vi "Set New Product.vi"(6 "error in (no error)":errorcluster, 9 "Cluster":T1) -> (0 "error out":errorcluster, 3 "success?":bool)   [LabVIEW 2020, in "SQLITE Inventory.lvlib"]
uses:
  SQLITE Inventory.lvlib
  Invetory Data Type.ctl
  <vilib>/drjdpowell/SQLite Library/SQL Connection/Open (path).vi
  <vilib>/drjdpowell/SQLite Library/SQL Connection/Open (string).vi
  <vilib>/AdvancedString/Path To Command Line String.vi
  <vilib>/drjdpowell/SQLite Library/SQL Connection/Execute SQL (No results).vi
  <vilib>/drjdpowell/SQLite Library/SQL Connection/Connection.lvclass
  <vilib>/drjdpowell/SQLite Library/SQLite.lvlib
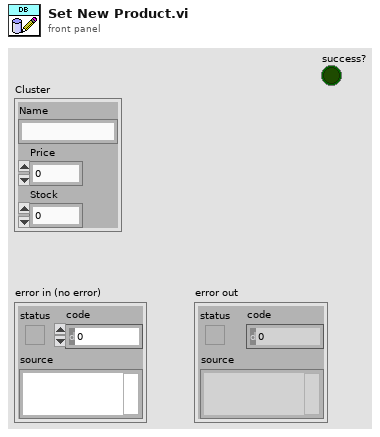
[diagram p1: front panel]
types:
  T1 = typedef "Invetory Data Type.ctl" = cluster{"Name":string, "Price":dbl, "Stock":dbl}
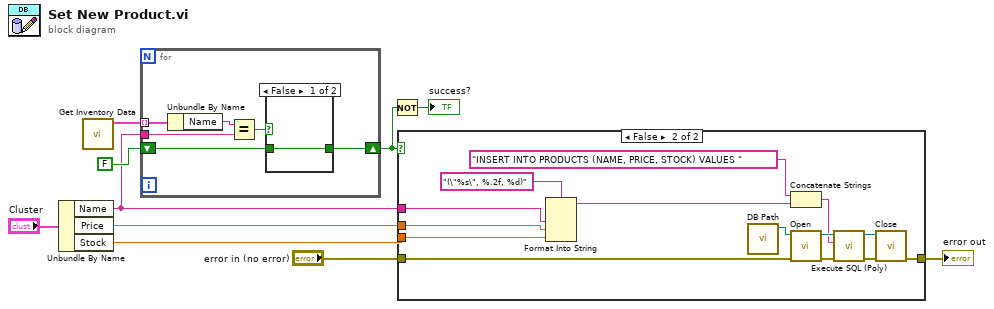
[diagram p0: block diagram]
diagram:
  n1 = Unbundle By Name("Cluster") -> ("Name"=w1:string, "Price"=w9:dbl, "Stock"=w8:dbl)
  n2 = call "Get Inventory Data.vi"() -> ("Array"=w7:T1[])  [unwired: 10 in, 1 out]
  n3 = for {
    tunnel: w7 -> [w15] mode=indexing
    tunnel: w1 -> [w16]
    shift-right: [w12] -> w3
    shift-left: FALSE -> [w11]
    n4 = Unbundle By Name(w15) -> ("Name"=w14:string)
    n5 = Equal?(x=w14, y=w16) -> (x = y?=w13:bool)
    n6 = case shown="False" w13 {
      selector: w13 -> [_ w18]
      tunnel: [w17 w18] -> w12
      tunnel: w11 -> [w17 _]
      frame False {
      }
      frame True {
      }
    }
  }
  n7 = Not(x=w3) -> (.not. x?=→"success?":bool)
  n8 = case shown="False" w3 {
    tunnel: w9 -> [_ w24]
    tunnel: w8 -> [_ w23]
    tunnel: "error in (no error)" -> [w19 w22]
    tunnel: [w19 w21] -> w4
    tunnel: w1 -> [_ w20]
    frame True {
    }
    frame False {
      n9 = Format Into String(format string="(\"%s\", %.2f, %d)", w20, w24, w23) -> (resulting string=w26:string)  [unwired: 2 in, 1 out]
      n10 = call "DB Path.vi"() -> ("DB Path"=w29:path)  [unwired: 11 in]
      n11 = Concatenate Strings("INSERT INTO PRODUCTS (NAME, PRICE, STOCK) VALUES " ("SQL"), w26) -> (w25:string)
      n12 = call-poly <vilib>:"Open.vi"("error in (no error)"=w22, "db file"=w29) -> ("error out"=w31:errorcluster, "SQLite Connection"=w33:refnum<class "Connection.lvclass">)  [unwired: 8 in]
      n13 = call-poly <vilib>:"Execute SQL (Poly).vi"("error in (no error)"=w31, "SQL"=w25, "SQLite Connection in"=w33) -> ("error out"=w30:errorcluster, "SQLite Connection"=w32:refnum<class "Connection.lvclass">)  [unwired: 7 in]
      n14 = call-dynamic "Close.vi"("error in (no error)"=w30, "SQLite Connection in"=w32) -> ("error out"=w21:errorcluster)  [unwired: 9 in]
    }
  }
  "error out" <- w4
